vi "Configure Trigger.vi"(8 "error in (no error)":errorcluster, 9 "Trigger Time":dbl=999.99 min=0.01 max=999.99, 10 "Trigger Source 0:BUS":u16(ring) items=["BUS", "External", "HOLD", "Manual", "Timer"], 11 "VISA resource name":refnum<visa-resource-name>) -> (0 "error out":errorcluster, 3 "VISA resource name out":refnum<visa-resource-name>)   [LabVIEW 2015, in "IT8900A-E.lvlib"]
doc: "This command selects the trigger source and internal trigger source generation trigger cycles.\n<b>Trigger Source</b>\n0:<b>BUS</b>:Accept a GPIB <GET> signal or a *TRG command as the trigger source, which ensures that all current commands complete before triggering occurs.\n1:<b>EXT</b>:Select electronic load input as the trigger source.Once received, the trigger is processed.\n2:<b>HOLD</b>:Only the TRIG:IMM command will generate a trigger in HOLD mode.All other trigger commands are not considered.\n3:<b>MANU</b>:This event occurs when the Trig key is pressed.\n4:<b>TIM</b>:The generation trigger synchronizes with the crystal vibration within the electronic load as the trigger source.As soon as the command is executed, the synchronous vibration starts to run.Edit the vibration cycle using TRIG:TIM.\n\nDefault:0 BUS Mode."
uses:
  <instrlib>/IT8900/IT8900A-E.lvlib
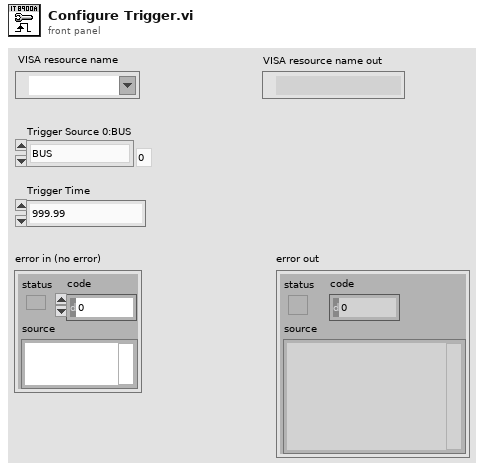
[diagram p1: front panel]
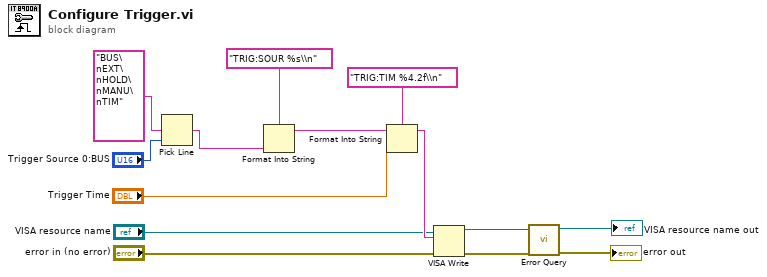
[diagram p0: block diagram]
diagram:
  n1 = Pick Line(multi-line string="BUS\nEXT\nHOLD\nMANU\nTIM", line index="Trigger Source 0:BUS") -> (output string=w1:string)  [unwired: 1 in]
  n2 = Format Into String(format string="TRIG:SOUR %s\\n", w1) -> (resulting string=w11:string)  [unwired: 2 in, 1 out]
  n3 = Format Into String(format string="TRIG:TIM %4.2f\\n", initial string=w11, "Trigger Time") -> (resulting string=w10:string)  [unwired: 1 in, 1 out]
  n4 = VISA Write(VISA resource name="VISA resource name", write buffer=w10, error in (no error)="error in (no error)") -> (VISA resource name out=w7:refnum<visa-resource-name>, error out=w6:errorcluster)  [unwired: 1 out]
  n5 = call <instrlib>:"Error Query.vi"("error in (no error)"=w6, "VISA resource name"=w7) -> ("error out"=→"error out":errorcluster, "VISA resource name out"=→"VISA resource name out":refnum<visa-resource-name>)  [unwired: 6 in, 2 out]
